vi "push_nil.vi"(8 "error in (no error)":errorcluster, 10 "ignored":bool, 11 "Lua in":refnum<class "Lua.lvclass">) -> (0 "error out":errorcluster, 3 "Lua out":refnum<class "Lua.lvclass">)   [LabVIEW 2020, in "Lua for LabVIEW.lvlib" / "Lua.lvclass"]
doc: "Push a nil value to the Lua stack (boolean input value is ignored)."
uses:
  Lua.lvclass
  Lua.lvclass/Lua.ctl
  lib/lua.dll/lua.dll.lvlib
  lib/lua.dll/lua_pushnil.vi
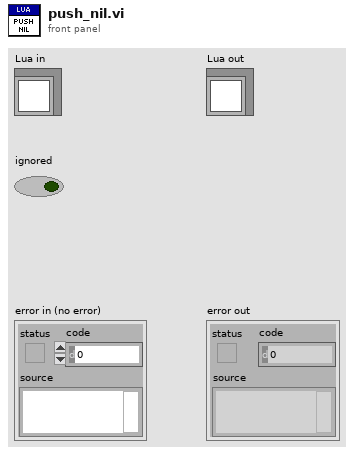
[diagram p1: front panel]
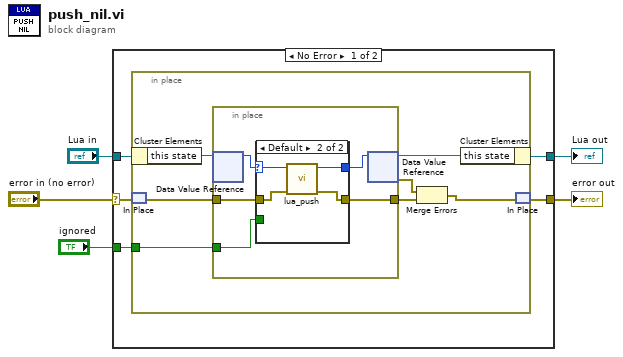
[diagram p0: block diagram]
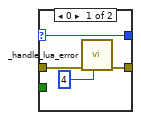
[diagram p2: hidden frame]
diagram:
  n1 = case shown="No Error" "error in (no error)" {
    selector: "error in (no error)" -> [w7 w32]
    tunnel: [w8 w32] -> w4
    tunnel: [w9 w31] -> w2
    tunnel: "Lua in" -> [w10 w31]
    tunnel: "ignored" -> [w6 _]
    frame No Error {
      n2 = in-place {
        in-place-border: w6 -> [w16]
        n3 = in-place-cluster #1(w10) -> ("this state"=w14:refnum<data-value>)
        n4 = in-place-match #2(w7) -> (w17:errorcluster)
        n5 = in-place {
          in-place-border: w17 -> [w22]
          in-place-border: w16 -> [w21]
          in-place-border: [w18] -> w12
          n6 = in-place-dvr #3(w14) -> (w19:u64)  [unwired: 1 out]
          n7 = case shown="Default" w19 {
            selector: w19 -> [w26 w29]
            tunnel: [w26 w30] -> w20
            tunnel: w22 -> [w23 w28]
            tunnel: [w24 w27] -> w18
            tunnel: w21 -> [_ _]
            frame 0 {
              n8 = call "_handle_lua_error.vi"("lua status"=4 ("lua_load errcode"), "error in (no error)"=w23) -> ("error out"=w24:errorcluster)  [unwired: 9 in]
            }
            frame Default {
              n9 = call-poly "lua_push.vi"("error in (no error)"=w28, "lua_state_p"=w29) -> ("error out"=w27:errorcluster, "lua_state_p out"=w30:u64)  [unwired: 8 in]
            }
          }
          n10 = in-place-dvr #3(w20) -> (w15:refnum<data-value>, w13:errorcluster)
        }
        n11 = Merge Errors(w13, w12) -> (w11:errorcluster)
        n12 = in-place-cluster #1("this state"=w15) -> (w9:refnum<class "Lua.lvclass">)
        n13 = in-place-match #2(w11) -> (w8:errorcluster)
      }
    }
    frame Error {
    }
  }
  "error out" <- w4
  "Lua out" <- w2
